vi "Insert VI into SubPanel.vi"(7 "AllowOpenBD":bool=TRUE, 8 "error in":errorcluster, 10 "SubPnl Ref":refnum<vi>, 11 "VI Ref":refnum<vi>) -> (0 "error out":errorcluster, 3 "Inserted VI's Name":string)   [LabVIEW 2025, in "Common Helpers.lvlib"]
uses:
  Common Helpers.lvlib
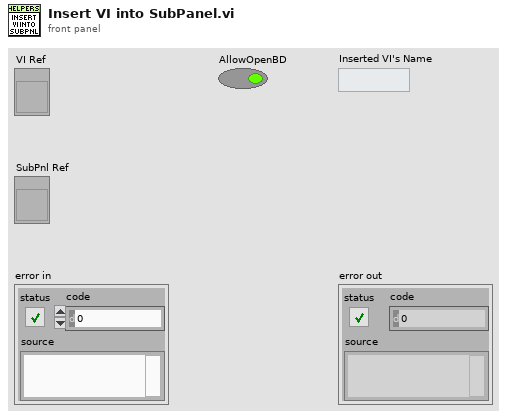
[diagram p1: front panel]
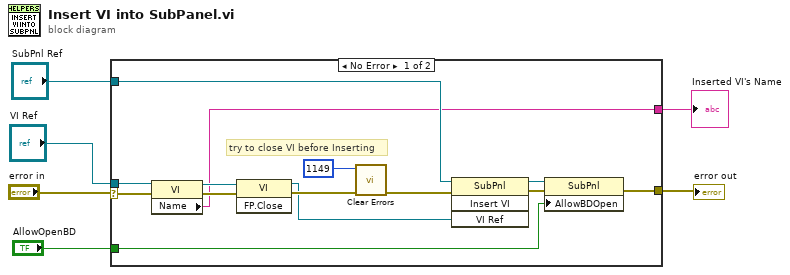
[diagram p0: block diagram]
diagram:
  n1 = case shown="No Error" "error in" {
    selector: "error in" -> [w15 w21]
    tunnel: "VI Ref" -> [w9 _]
    tunnel: [w14 w21] -> w5
    tunnel: "SubPnl Ref" -> [w16 _]
    tunnel: "AllowOpenBD" -> [w12 _]
    tunnel: [w7 _] -> w1
    frame No Error {
      # "try to close VI before Inserting"
      n2 = property class="VI"(reference=w9, error in=w15) -> (reference out=w8:refnum<vi>, error out=w10:errorcluster, "Name"=w7:string)
      n3 = invoke class="VI" method="FP.Close"(reference=w8, error in=w10) -> (reference out=w11:refnum<vi>, error out=w19:errorcluster)  [unwired: 1 in, 1 out]
      n4 = call <vilib>:"Clear Errors.vi"("error in (no error)"=w19, "specific error code to clear (0: all)"=1149) -> ("error out"=w18:errorcluster)  [unwired: 4 in, 1 out]
      n5 = invoke on="Invoke Node" class="SubPnl" method="Insert VI"(reference=w16, error in=w18, "VI Ref"=w11) -> (reference out=w13:refnum<vi>, error out=w17:errorcluster)  [unwired: 1 in, 2 out]
      n6 = property class="SubPnl"(reference=w13, error in=w17, "AllowBDOpen"=w12) -> (error out=w14:errorcluster)  [unwired: 1 out]
    }
    frame Error {
    }
  }
  "error out" <- w5
  "Inserted VI's Name" <- w1
